vi "Find VI in ProjectItem (DFS).vi"(8 "Error In":errorcluster, 10 "VI Filename (including extension)":string, 11 "Project Item Ref":refnum<vi>) -> (0 "Error Out":errorcluster, 3 "Search Output":T1)   [LabVIEW 2022 SP3]
doc: "This VI implements a Depth First Search (DFS) that searches for a given VI inside a LabVIEW Project (lvproj), a project library (lvlib) or a class (lvclass).\n\nInputs:\n1. ProjectItem reference. This could be the reference of a LabVIEW Project (lvproj), a project library (lvlib) or a class (lvclass).\n\n2. VI filename (including extension). E.g. \"my VI.vi\"\n\nOutputs:\nA typedef cluster that contains the following information:\n - Whether the VI was found or not inside the given ProjectItem\nIf the VI was found:\n - The ProjectItem reference of the VI\n - The ProjectItem reference of the owning virtual folder (if any)\n - A string that represents the virtual folder path. E.g. \"folder 1\\folder2\\folder 3\"\n\nThe search automatically aborts if a certain maximum allowed amount of time has elapsed (e.g. two seconds). This search executes as part of the app launch. If the search takes too long the app will launch sluggishly. That's why we want to limit the maximum search time."
uses:
  DFS Node (cluster).ctl
  DFS Child Node (cluster).ctl
  DFS States (enum).ctl
  DFS Output (cluster).ctl
panel:
  out "No. of executions\nGet Index Of Next Node To Search":i32
  out "Execution Duration (ms)":u32
  out "Number of states":i32
  out "Found Node Index":i32
  out "States":T2[](array[typedef])
  out "DFS Node Found (Dev Indicator)":T3
  out "Loop Iteration":i32
  # "Development\nControls or indicators that are useful for development or testing, but which are not outputs of the VI."
  # "Input\nInputs to the VI"
  # "Output\nOutputs of the VI"
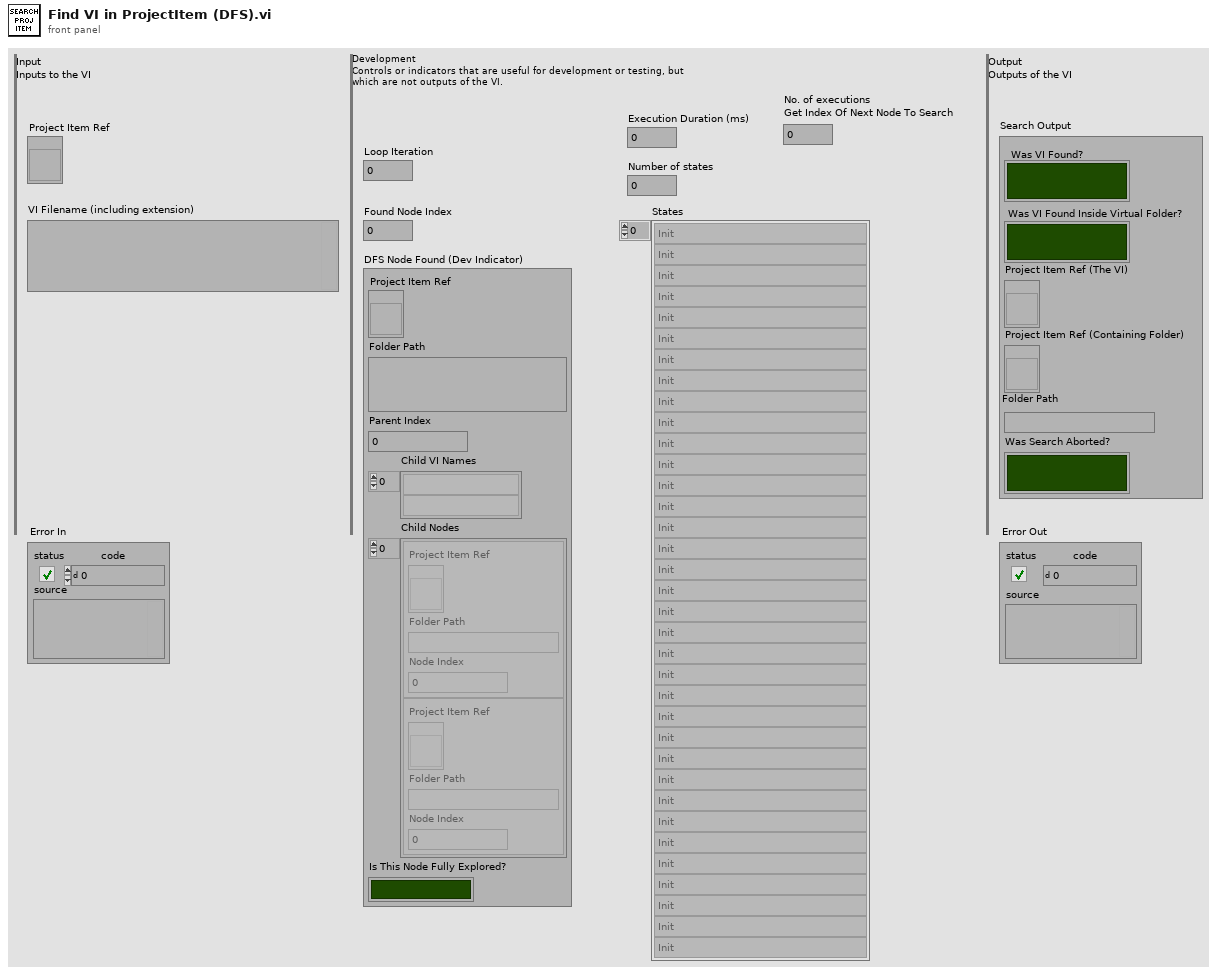
[diagram p1: front panel]
types:
  T1 = typedef "DFS Output (cluster).ctl" = cluster{"Was VI Found?":bool, "Was VI Found Inside Virtual Folder?":bool, "Project Item Ref (The VI)":refnum<vi>, "Project Item Ref (Containing Folder)":refnum<vi>, "Folder Path":string, "Was Search Aborted?":bool}
  T2 = typedef "DFS States (enum).ctl" = enum16{"Init", "Add Children", "Search For VI", "Get Index Of Next Node To Search", "VI Was Found", "VI Was Not Found", "Allowed Execution Time Has Elapsed"}
  T3 = typedef "DFS Node (cluster).ctl" = cluster{"Project Item Ref":refnum<vi>, "Folder Path":string, "Parent Index":i32, "Child VI Names":string[], "Child Nodes":T4[], "Is This Node Fully Explored?":bool}
  T4 = typedef "DFS Child Node (cluster).ctl" = cluster{"Project Item Ref":refnum<vi>, "Folder Path":string, "Node Index":i32}
  T5 = typedef "DFS Data (cluster).ctl" = cluster{"Current Index":i32, "ProjectItem Ref Of Searched VI":refnum<vi>, "Nodes":T3[]}
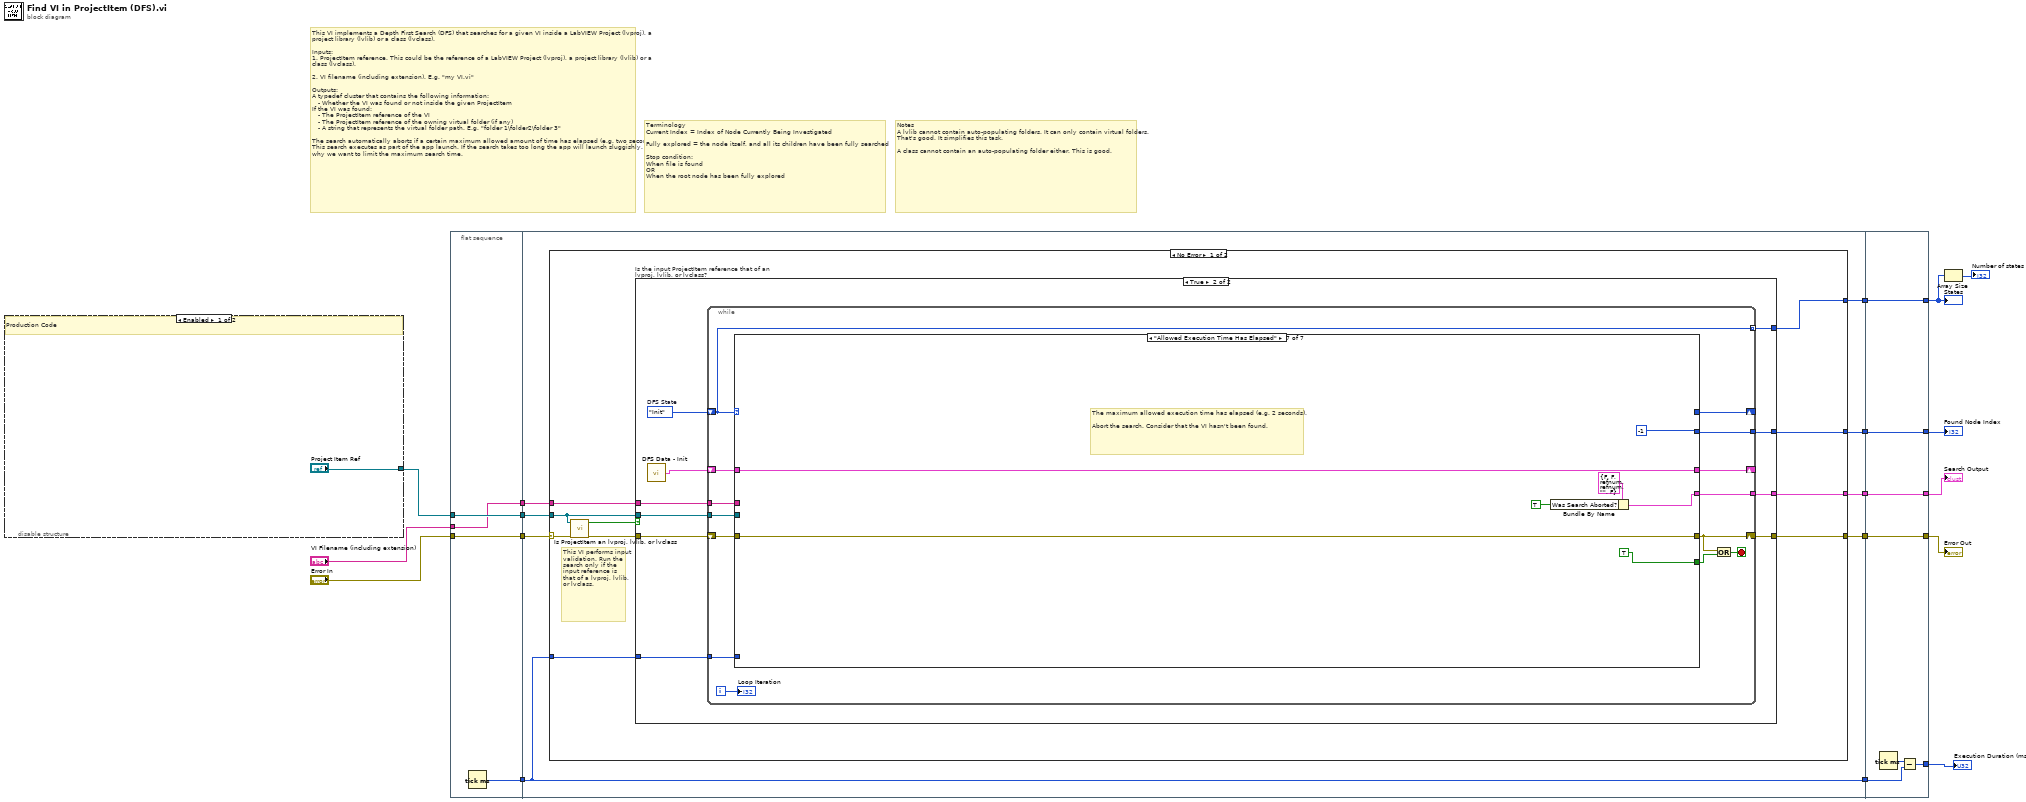
[diagram p0: block diagram]
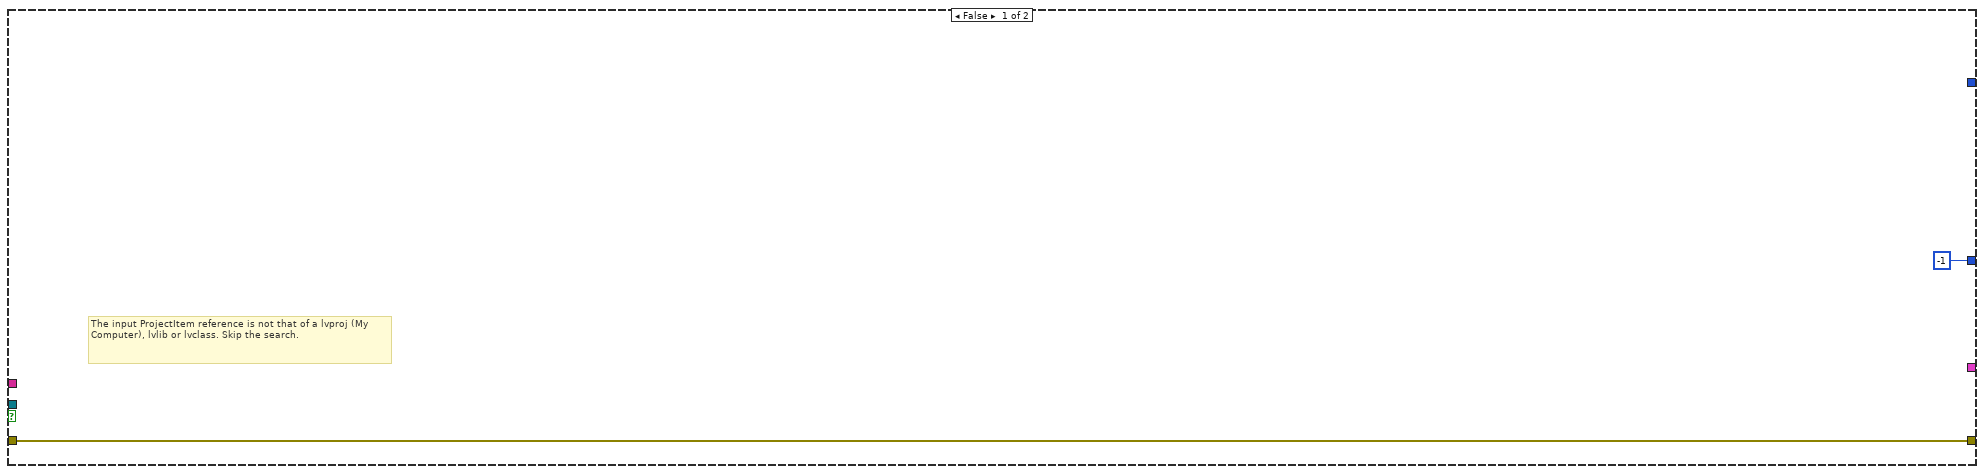
[diagram p2: hidden frame]
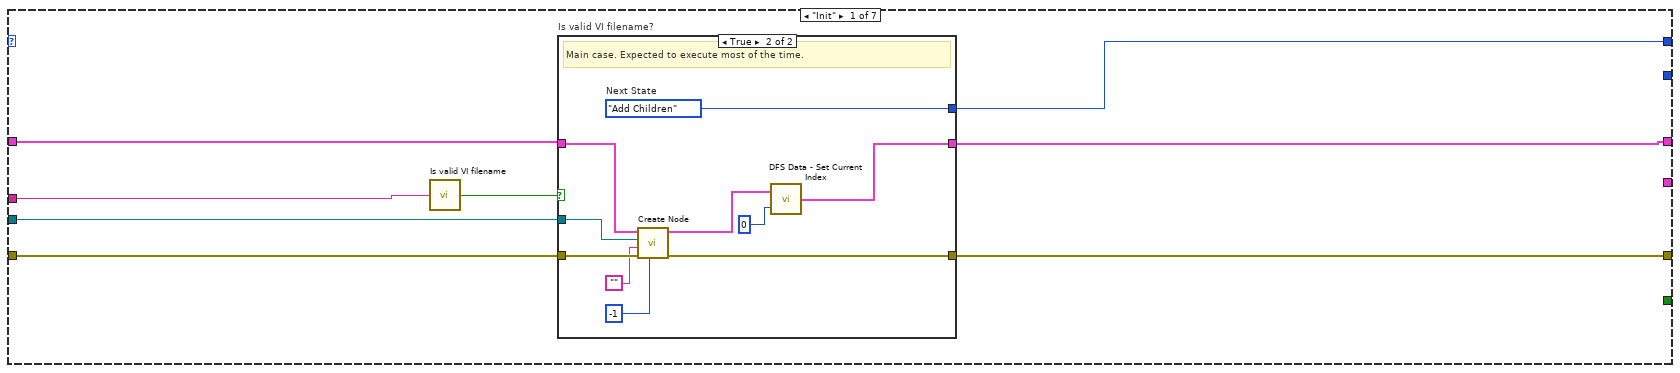
[diagram p3: hidden frame]
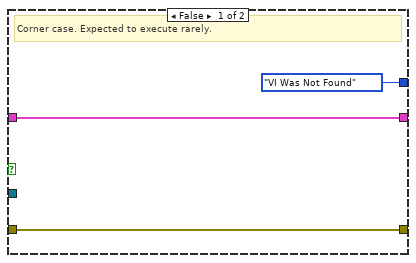
[diagram p4: hidden frame]
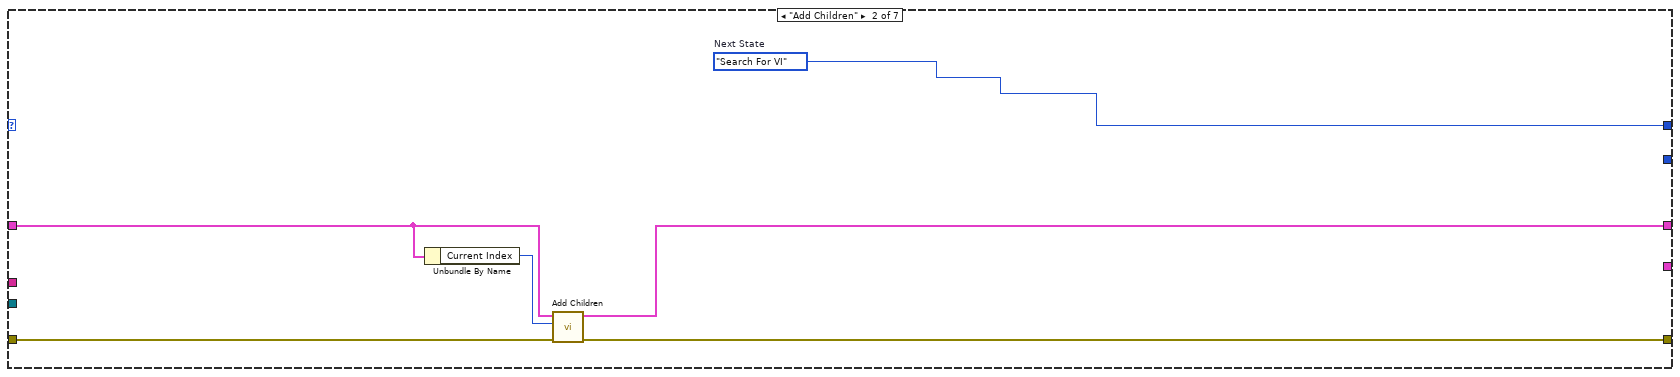
[diagram p5: hidden frame]
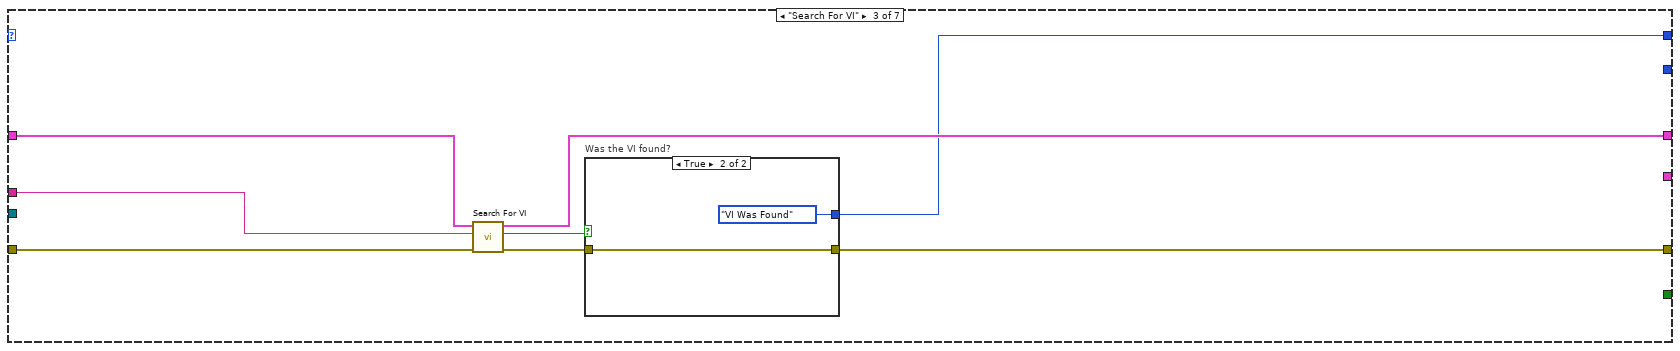
[diagram p6: hidden frame]
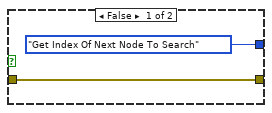
[diagram p7: hidden frame]
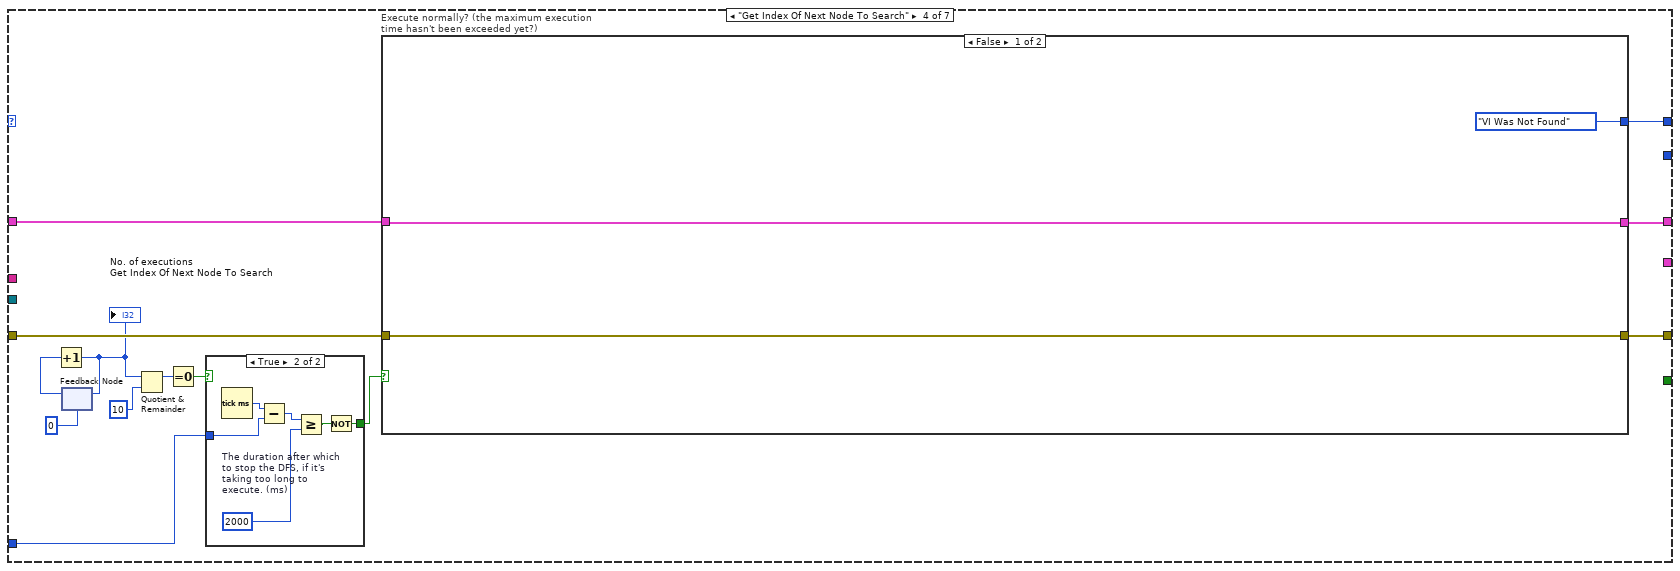
[diagram p8: hidden frame]
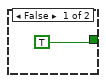
[diagram p9: hidden frame]
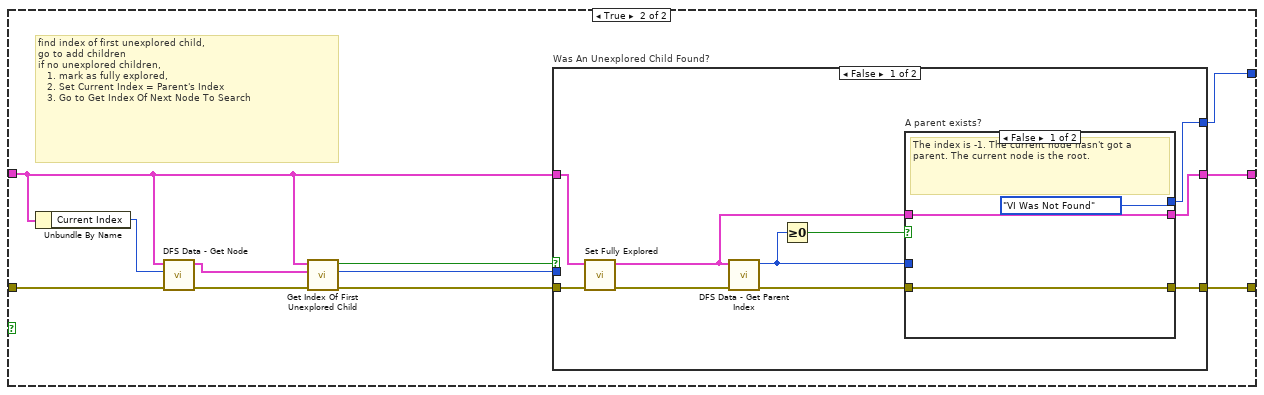
[diagram p10: hidden frame]
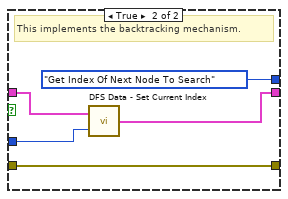
[diagram p11: hidden frame]
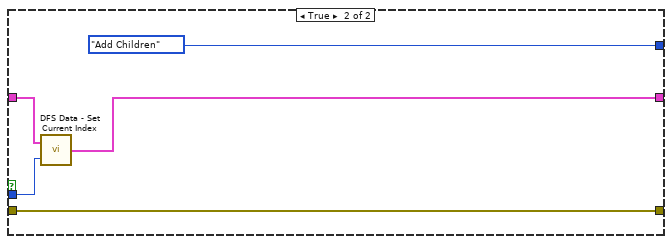
[diagram p12: hidden frame]
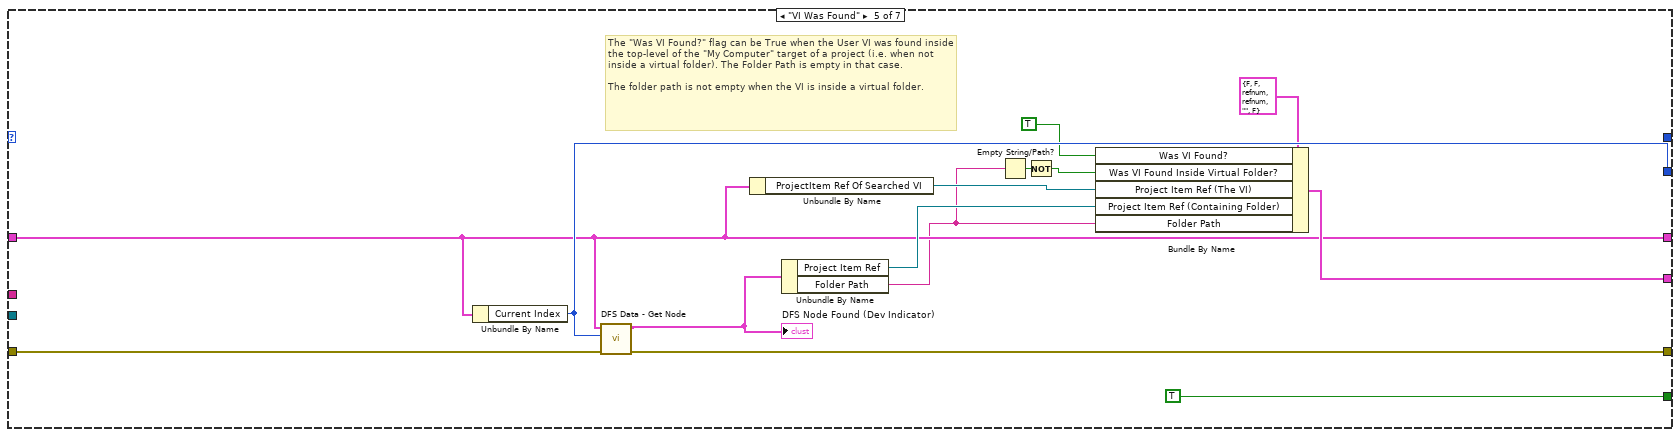
[diagram p13: hidden frame]
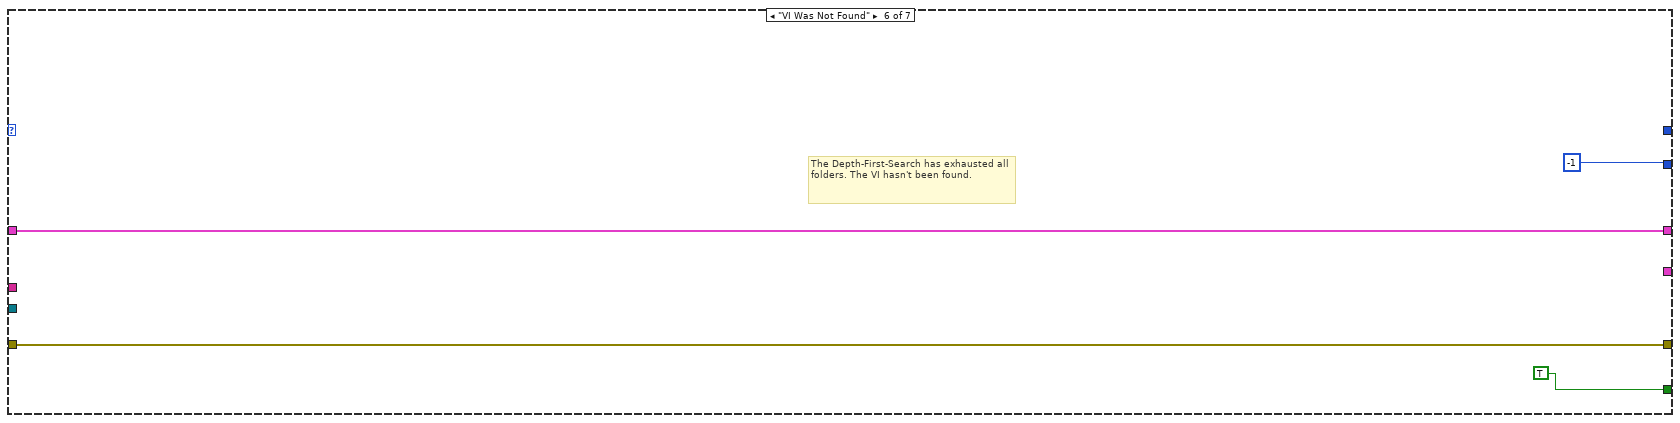
[diagram p14: hidden frame]
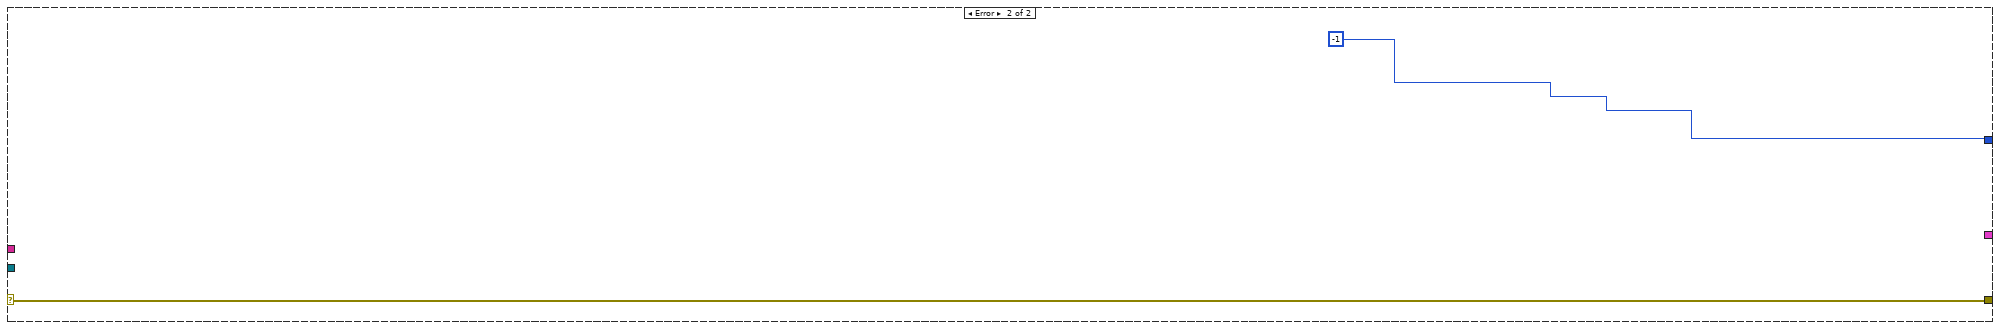
[diagram p15: hidden frame]
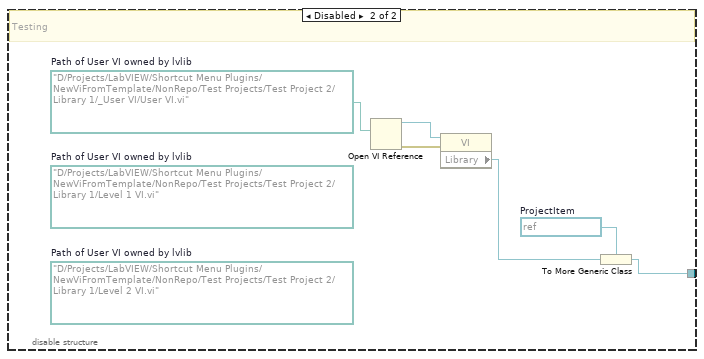
[diagram p16: hidden frame]
diagram:
  # "Notes\nA lvlib cannot contain auto-populating folders. It can only contain virtual folders. That's good. It simplifies this task.\n\nA class cannot contain an auto-populating folder either. This is good."
  # "Terminology\nCurrent Index = Index of Node Currently Being Investigated\n\nFully explored = the node itself, and all its children have been fully searched\n\nStop condition:\nWhen file is found\nOR\nWhen the root node has been fully explored"
  # "This VI implements a Depth First Search (DFS) that searches for a given VI inside a LabVIEW Project (lvproj), a project library (lvlib) or a class (lvclass).\n\nInputs:\n1. ProjectItem reference. This could be the reference of a LabVIEW Project (lvproj), a project library (lvlib) or a class (lvclass).\n\n2. VI filename (including extension). E.g. \"my VI.vi\"\n\nOutputs:\nA typedef cluster that contains the following information:\n   - Whether the VI was found or not inside the given ProjectItem\nIf the VI was found:\n   - The ProjectItem reference of the VI\n   - The ProjectItem reference of the owning virtual folder (if any)\n   - A string that represents the virtual folder path. E.g. \"folder 1\\folder2\\folder 3\"\n\nThe search automatically aborts if a certain maximum allowed amount of time has elapsed (e.g. two seconds). This search executes as part of the app launch. If the search takes too long the app will launch sluggishly. That's why we want to limit the maximum search time."
  n1 = disable-structure shown="Enabled" {
    disable-tunnel: ["Project Item Ref" w20] -> w16
    frame Enabled {
      # "Production Code"
    }
    frame Disabled {
      w21 = refnum<vi> refnum  # ProjectItem
      (unwired) path "D:/Projects/LabVIEW/Shortcut Menu Plugins/NewViFromTemplate/NonRepo/Test Projects/Test Project 2/Library 1/Level 2 VI.vi"  # Path of User VI owned by lvlib
      (unwired) path "D:/Projects/LabVIEW/Shortcut Menu Plugins/NewViFromTemplate/NonRepo/Test Projects/Test Project 2/Library 1/Level 1 VI.vi"  # Path of User VI owned by lvlib
      w25 = path "D:/Projects/LabVIEW/Shortcut Menu Plugins/NewViFromTemplate/NonRepo/Test Projects/Test Project 2/Library 1/_User VI/User VI.vi"  # Path of User VI owned by lvlib
      # "Testing"
      n2 = Open VI Reference(vi path=w25) -> (vi reference=w23:refnum<vi>, error out=w24:errorcluster)  [unwired: 5 in]
      n3 = property class="VI"(reference=w23, error in=w24) -> ("Library"=w22:refnum<vi>)  [unwired: 2 out]
      n4 = To More Generic Class(target class=w21, reference=w22) -> (generic class reference=w20:refnum<vi>)
    }
  }
  n5 = flat-sequence {
    tunnel: "VI Filename (including extension)" -> [w27]
    tunnel: w16 -> [w28]
    tunnel: "Error In" -> [w29]
    tunnel: [w29] -> w13
    tunnel: [w28] -> w12
    tunnel: [w27] -> w11
    tunnel: [w26] -> w8
    tunnel: w13 -> [w37]
    tunnel: w12 -> [w35]
    tunnel: w11 -> [w34]
    tunnel: [w36] -> w10
    tunnel: [w33] -> w9
    tunnel: w8 -> [w30]
    tunnel: [w30] -> w7
    tunnel: [w32] -> w4
    tunnel: [w31] -> w1
    tunnel: [w202] -> w15
    tunnel: [w203] -> w17
    tunnel: w10 -> [w203]
    tunnel: w9 -> [w202]
    tunnel: w7 -> [w200]
    tunnel: [w199] -> w6
    tunnel: [w198] -> w5
    tunnel: w4 -> [w198]
    tunnel: [w197] -> w2
    tunnel: w1 -> [w197]
    frame #0 {
      n6 = Tick Count (ms)() -> (millisecond timer value=w26:u32)
    }
    frame #1 {
      n7 = case shown="No Error" w37 {
        selector: w37 -> [w41 w196]
        tunnel: [w47 w196] -> w36
        tunnel: w35 -> [w39 _]
        tunnel: w34 -> [w46 _]
        tunnel: [w45 _] -> w33
        tunnel: [w44 -1 ("Current Index")] -> w32
        tunnel: [w43 _] -> w31
        tunnel: w30 -> [w42 _]
        frame No Error {
          # "This VI performs input validation. Run the search only if the input reference is that of a lvproj, lvlib, or lvclass."
          n8 = call "Is ProjectItem an lvproj, lvlib, or lvclass.vi"("Error In"=w41, "Project Item Ref"=w39) -> ("Error Out"=w40:errorcluster, "Is the input ProjectItem reference that of an lvproj, lvlib, or lvclass?"=w38:bool)  [unwired: 8 in]
          n9 = case "Is the input ProjectItem reference that of an lvproj, lvlib, or lvclass?" shown="True" w38 {
            tunnel: w40 -> [w49 w58]
            tunnel: [w49 w57] -> w47
            tunnel: w39 -> [_ w56]
            tunnel: w46 -> [_ w54]
            tunnel: [_ w53] -> w45
            tunnel: [-1 ("Current Index") w52] -> w44
            tunnel: [_ w51] -> w43
            tunnel: w42 -> [_ w50]
            frame False {
              # "The input ProjectItem reference is not that of a lvproj (My Computer), lvlib or lvclass. Skip the search."
            }
            frame True {
              w59 = DFS_States_(enum)."Init"  # DFS State
              n10 = call "DFS Data - Init.vi"() -> ("Initial DFS Data"=w55:T5)
              n11 = while {
                shift-right: [w66] -> _
                shift-left: w59 -> [w63]
                shift-right: [w67] -> w57
                shift-left: w58 -> [w73]
                shift-right: [w69] -> _
                shift-left: w55 -> [w71]
                tunnel: w56 -> [w70]
                tunnel: w54 -> [w65]
                tunnel: [w63] -> w53 mode=indexing
                tunnel: [w62] -> w52
                tunnel: [w61] -> w51
                tunnel: w50 -> [w60]
                i -> [w72]
                stop <- w68 stop-if-true
                n12 = case shown="\"Allowed Execution Time Has Elapsed\"" w63 {
                  tunnel: w73 -> [w81 w100 w108 w125 w183 w187 w194]
                  tunnel: [w76 w99 w103 w124 w182 w187 w194] -> w67
                  tunnel: w71 -> [w80 w96 w106 w122 w174 w186 w193]
                  tunnel: w70 -> [w79 _ _ _ _ _ _]
                  tunnel: [w78 w97 w105 w123 w174 w186 w193] -> w69
                  tunnel: [w77 w95 w101 w121 _ _ _] -> w66
                  tunnel: w65 -> [w75 _ w104 _ _ _ _]
                  tunnel: [_ _ _ _ TRUE TRUE TRUE] -> w64
                  tunnel: [_ _ _ _ w180 -1 ("Current Index") -1 ("Current Index")] -> w62
                  tunnel: [_ _ _ _ w175 _ w189] -> w61
                  tunnel: w60 -> [_ _ _ w114 _ _ _]
                  frame "Init" {
                    n13 = call "Is valid VI filename.vi"("VI Filename"=w75) -> ("Is VI filename valid?"=w74:bool)
                    n14 = case "Is valid VI filename?" shown="True" w74 {
                      tunnel: w81 -> [w82 w94]
                      tunnel: w80 -> [w83 w93]
                      tunnel: w79 -> [_ w92]
                      tunnel: [w83 w88] -> w78
                      tunnel: [DFS_States_(enum)."VI Was Not Found" ("Next State") w87] -> w77
                      tunnel: [w82 w85] -> w76
                      frame False {
                        # "Corner case. Expected to execute rarely."
                      }
                      frame True {
                        w87 = DFS_States_(enum)."Add Children"  # Next State
                        # "Main case. Expected to execute most of the time."
                        n15 = call "Create Node.vi"("Parent Index"=-1, "Error In"=w94, "Folder Path"="", "Project Item"=w92, "DFS Data In"=w93) -> ("Error Out"=w85:errorcluster, "DFS Data Out"=w86:T5)  [unwired: 5 in]
                        n16 = call "DFS Data - Set Current Index.vi"("Current Index"=0 ("Parent Index"), "DFS Data In"=w86) -> ("DFS Data Out"=w88:T5)
                      }
                    }
                  }
                  frame "Add Children" {
                    w95 = DFS_States_(enum)."Search For VI"  # Next State
                    n17 = Unbundle By Name(w96) -> ("Current Index"=w98:i32)
                    n18 = call "Add Children.vi"("Error In"=w100, "Parent Index"=w98, "DFS Data In"=w96) -> ("Error Out"=w99:errorcluster, "DFS Data Out"=w97:T5)  [unwired: 7 in]
                  }
                  frame "Search For VI" {
                    n19 = call "Search For VI.vi"("Error In"=w108, "VI Filename To Search For"=w104, "DFS Data In"=w106) -> ("Error Out"=w107:errorcluster, "VI Found?"=w102:bool, "DFS Data Out"=w105:T5)  [unwired: 5 in, 1 out]
                    n20 = case "Was the VI found?" shown="True" w102 {
                      tunnel: w107 -> [w110 w112]
                      tunnel: [w110 w112] -> w103
                      tunnel: [DFS_States_(enum)."Get Index Of Next Node To Search" ("Next State") DFS_States_(enum)."VI Was Found" ("Next State")] -> w101
                      frame False {
                      }
                      frame True {
                      }
                    }
                  }
                  frame "Get Index Of Next Node To Search" {
                    n21 = feedback #1(0) -> (w120:i32)
                    n22 = Increment(x=w120) -> (x+1=w118:i32)
                    "No. of executions\nGet Index Of Next Node To Search" <- w118
                    n23 = feedback-in #1(w118) -> ()
                    n24 = Quotient & Remainder(x=w118, y=10) -> (x-y*floor(x/y)=w116:i32)  [unwired: 1 out]
                    n25 = Equal To 0?(x=w116) -> (x = 0?=w115:bool)
                    n26 = case shown="True" w115 {
                      tunnel: w114 -> [_ w130]
                      tunnel: [TRUE w127] -> w113
                      frame False {
                      }
                      frame True {
                        w129 = u32 2000  # The duration after which to stop the DFS, if it's taking too long to execute. (ms)
                        n27 = Tick Count (ms)() -> (millisecond timer value=w131:u32)
                        n28 = Subtract(x=w131, y=w130) -> (x-y=w132:u32)
                        n29 = Greater Or Equal?(x=w132, y=w129) -> (x >= y?=w128:bool)
                        n30 = Not(x=w128) -> (.not. x?=w127:bool)
                      }
                    }
                    n31 = case "Execute normally? (the maximum execution time hasn't been exceeded yet?)" shown="False" w113 {
                      tunnel: w125 -> [w134 w144]
                      tunnel: [w134 w141] -> w124
                      tunnel: [w133 w138] -> w123
                      tunnel: w122 -> [w133 w137]
                      tunnel: [DFS_States_(enum)."VI Was Not Found" ("Next State") w136] -> w121
                      frame False {
                      }
                      frame True {
                        # "find index of first unexplored child,\ngo to add children\nif no unexplored children,\n   1. mark as fully explored,\n   2. Set Current Index = Parent's Index\n   3. Go to Get Index Of Next Node To Search"
                        n32 = Unbundle By Name(w137) -> ("Current Index"=w145:i32)
                        n33 = call "DFS Data - Get Node.vi"("Error In"=w144, "Node Index"=w145, "DFS Data"=w137) -> ("Error Out"=w143:errorcluster, "DFS Node"=w142:T3)  [unwired: 7 in]
                        n34 = call "Get Index Of First Unexplored Child.vi"("Error In"=w143, "DFS Node"=w142, "DFS Data"=w137) -> ("Error Out"=w146:errorcluster, "Index Of First Unexplored Child"=w139:i32, "Was An Unexplored Child Found?"=w140:bool)  [unwired: 6 in]
                        n35 = case "Was An Unexplored Child Found?" shown="False" w140 {
                          tunnel: w146 -> [w156 w169]
                          tunnel: [w152 w169] -> w141
                          tunnel: w139 -> [_ w168]
                          tunnel: [w147 w167] -> w138
                          tunnel: w137 -> [w154 w166]
                          tunnel: [w150 DFS_States_(enum)."Add Children" ("Next State")] -> w136
                          frame False {
                            n36 = call "Set Fully Explored.vi"("Error In"=w156, "DFS Data In"=w154) -> ("Error Out"=w155:errorcluster, "DFS Data Out"=w148:T5)  [unwired: 8 in]
                            n37 = call "DFS Data - Get Parent Index.vi"("Error In"=w155, "DFS Data In"=w148) -> ("Error Out"=w153:errorcluster, "Parent Index"=w149:i32)  [unwired: 8 in]
                            n38 = Greater Or Equal To 0?(x=w149) -> (x >= 0?=w151:bool)
                            n39 = case "A parent exists?" shown="False" w151 {
                              tunnel: w153 -> [w159 w164]
                              tunnel: [w159 w164] -> w152
                              tunnel: [DFS_States_(enum)."VI Was Not Found" ("Next State") DFS_States_(enum)."Get Index Of Next Node To Search" ("Next State")] -> w150
                              tunnel: w149 -> [_ w162]
                              tunnel: w148 -> [w157 w161]
                              tunnel: [w157 w160] -> w147
                              frame False {
                                # "The index is -1. The current node hasn't got a parent. The current node is the root."
                              }
                              frame True {
                                # "This implements the backtracking mechanism."
                                n40 = call "DFS Data - Set Current Index.vi"("Current Index"=w162, "DFS Data In"=w161) -> ("DFS Data Out"=w160:T5)
                              }
                            }
                          }
                          frame True {
                            n41 = call "DFS Data - Set Current Index.vi"("Current Index"=w168, "DFS Data In"=w166) -> ("DFS Data Out"=w167:T5)
                          }
                        }
                      }
                    }
                  }
                  frame "VI Was Found" {
                    # "The \"Was VI Found?\" flag can be True when the User VI was found inside the top-level of the \"My Computer\" target of a project (i.e. when not inside a virtual folder). The Folder Path is empty in that case.\n\nThe folder path is not empty when the VI is inside a virtual folder."
                    n42 = Unbundle By Name(w174) -> ("Current Index"=w180:i32)
                    n43 = call "DFS Data - Get Node.vi"("Error In"=w183, "Node Index"=w180, "DFS Data"=w174) -> ("Error Out"=w182:errorcluster, "DFS Node"=w176:T3)  [unwired: 7 in]
                    "DFS Node Found (Dev Indicator)" <- w176
                    n44 = Unbundle By Name(w174) -> ("ProjectItem Ref Of Searched VI"=w173:refnum<vi>)
                    n45 = Unbundle By Name(w176) -> ("Project Item Ref"=w178:refnum<vi>, "Folder Path"=w171:string)
                    n46 = Empty String/Path?(string/path=w171) -> (empty?=w172:bool)
                    n47 = Not(x=w172) -> (.not. x?=w170:bool)
                    n48 = Bundle By Name(cluster=T1 {"Was VI Found?"=FALSE, "Was VI Found Inside Virtual Folder?"=FALSE, "Project Item Ref (The VI)"=refnum, "Project Item Ref (Containing Folder)"=refnum, "Folder Path"="", "Was Search Aborted?"=FALSE} ("DFS Output"), "Was VI Found?"=TRUE ("Was File Found?"), "Was VI Found Inside Virtual Folder?"=w170, "Project Item Ref (The VI)"=w173, "Project Item Ref (Containing Folder)"=w178, "Folder Path"=w171) -> (w175:T1)
                  }
                  frame "VI Was Not Found" {
                    # "The Depth-First-Search has exhausted all folders. The VI hasn't been found."
                  }
                  frame "Allowed Execution Time Has Elapsed" {
                    # "The maximum allowed execution time has elapsed (e.g. 2 seconds).\n\nAbort the search. Consider that the VI hasn't been found."
                    n49 = Bundle By Name(cluster=T1 {"Was VI Found?"=FALSE, "Was VI Found Inside Virtual Folder?"=FALSE, "Project Item Ref (The VI)"=refnum, "Project Item Ref (Containing Folder)"=refnum, "Folder Path"="", "Was Search Aborted?"=FALSE} ("DFS Output"), "Was Search Aborted?"=TRUE) -> (w189:T1)
                  }
                }
                n50 = Or(x=w67, y=w64) -> (x .or. y?=w68:bool)
                "Loop Iteration" <- w72
              }
            }
          }
        }
        frame Error {
        }
      }
    }
    frame #2 {
      n51 = Tick Count (ms)() -> (millisecond timer value=w201:u32)
      n52 = Subtract(x=w201, y=w200) -> (x-y=w199:u32)
    }
  }
  n53 = Array Size(array=w15) -> (size(s)=→"Number of states":i32)
  "Error Out" <- w17
  "States" <- w15
  "Execution Duration (ms)" <- w6
  "Found Node Index" <- w5
  "Search Output" <- w2
